vi "Finalize To Settings.vi"(8 "error in (no error)":errorcluster, 11 "Core Threads Configuration in":refnum<class "Thread Configuration.lvclass">) -> (0 "error out":errorcluster, 2 "settings":cluster{"key":string, "value":string}[](array[cluster]), 3 "Core Threads Configuration out":refnum<class "Thread Configuration.lvclass">)   [LabVIEW 2017, in "DSF Core.lvlib" / "Thread Configuration.lvclass"]
uses:
  Thread Configuration.lvclass
  Thread Configuration.lvclass/Thread Configuration.ctl
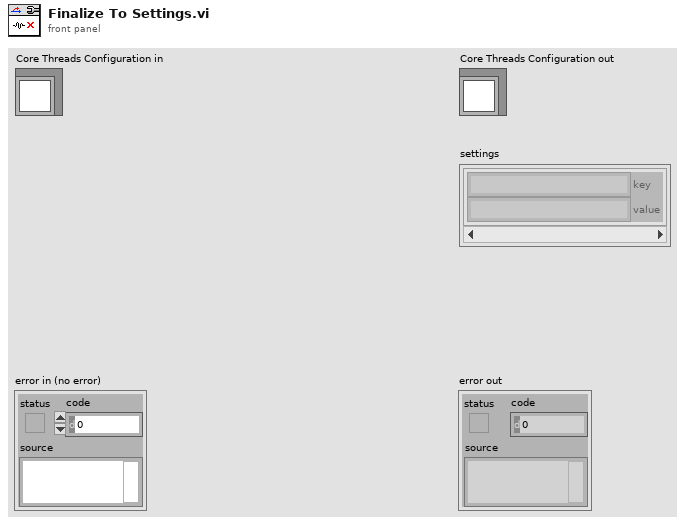
[diagram p1: front panel]
types:
  T1 = typedef "DSF Core.lvlib/Thread Configuration.lvclass/Core Thread Configuration.ctl" = cluster{"processor":i32, "priority offset":i16}
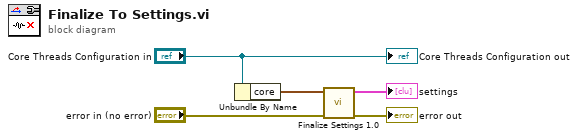
[diagram p0: block diagram]
diagram:
  n1 = Unbundle By Name("Core Threads Configuration in") -> ("core"=w3:T1)
  n2 = call "Finalize Settings 1.0.vi"("error in (no error)"="error in (no error)", "configuration 1.0"=w3) -> ("error out"=→"error out":errorcluster, "settings 1.0"=→"settings":cluster{"key":string, "value":string}[])  [unwired: 7 in, 1 out]
  "Core Threads Configuration out" <- "Core Threads Configuration in"
